vi "Pause.vi"(8 "error in (no error)":errorcluster, 11 "SSI PR Settings":T1) -> (0 "error out":errorcluster, 3 "SSI PR Settings":T1)   [LabVIEW 2018, in "SSI PR Pump.lvlib"]
uses:
  SSI PR Pump.lvlib
  SSI PR Settings Cluster.ctl
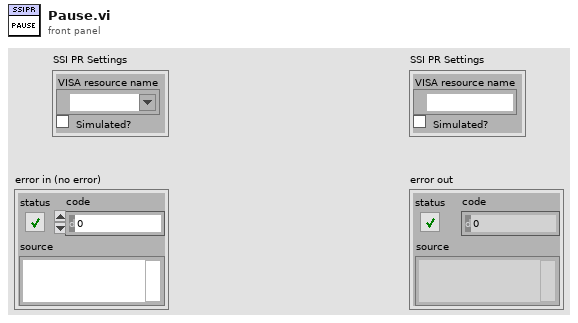
[diagram p1: front panel]
types:
  T1 = typedef "SSI PR Pump.lvlib/SSI PR Settings Cluster.ctl" = cluster{"VISA resource name":refnum<visa-resource-name>, "Simulated?":bool}
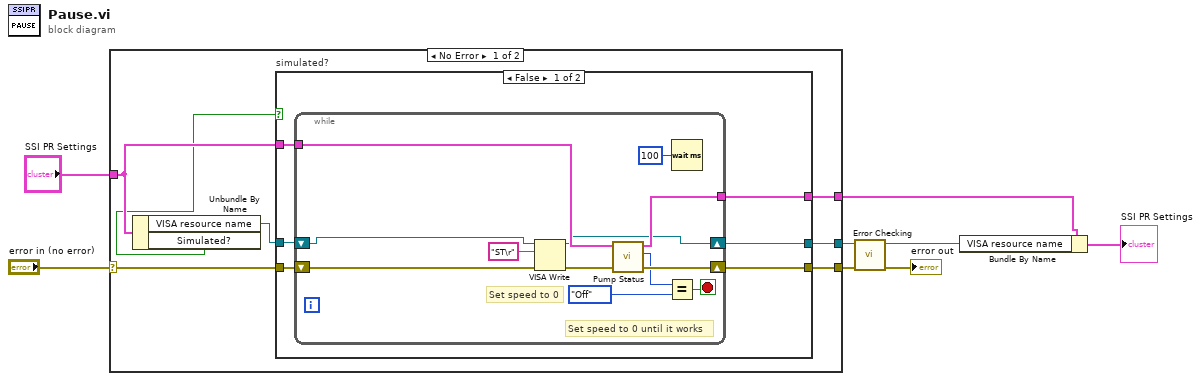
[diagram p0: block diagram]
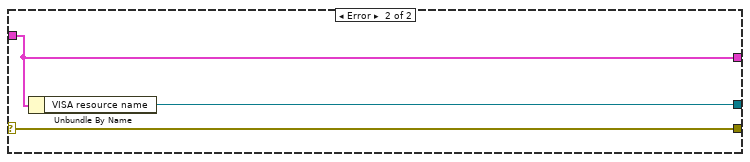
[diagram p3: hidden frame]
diagram:
  n1 = case shown="No Error" "error in (no error)" {
    selector: "error in (no error)" -> [w15 w39]
    tunnel: [w11 w38] -> w4
    tunnel: "SSI PR Settings" -> [w12 w38]
    tunnel: [w14 w37] -> w8
    tunnel: [w13 w39] -> w7
    frame No Error {
      n2 = Unbundle By Name(w12) -> ("VISA resource name"=w9:refnum<visa-resource-name>, "Simulated?"=w10:bool)
      n3 = case "simulated?" shown="False" w10 {
        tunnel: [w19 w36] -> w14
        tunnel: w9 -> [w21 w36]
        tunnel: w15 -> [w20 w35]
        tunnel: [w18 w35] -> w13
        tunnel: w12 -> [w17 w34]
        tunnel: [w16 w34] -> w11
        frame False {
          n4 = while {
            shift-right: [w23] -> w19
            shift-left: w21 -> [w33]
            shift-right: [w26] -> w18
            shift-left: w20 -> [w32]
            tunnel: w17 -> [w24]
            tunnel: [w25] -> w16
            stop <- w29 stop-if-true
            # "Set speed to 0 until it works"
            # "Set speed to 0"
            n5 = VISA Write(VISA resource name=w33, write buffer="ST\r" ("string"), error in (no error)=w32) -> (VISA resource name out=w23:refnum<visa-resource-name>, error out=w27:errorcluster)  [unwired: 1 out]
            n6 = call "Pump Status.vi"("error in (no error)"=w27, "SSI PR Settings"=w24) -> ("error out"=w26:errorcluster, "Pump On?"=w22:enum16{"Off", "On", "Not Initialized"}, "SSI PR Settings"=w25:T1)  [unwired: 5 in, 2 out]
            n7 = Equal?(x=w22, y=enum16{"Off", "On", "Not Initialized"}."Off") -> (x = y?=w29:bool)
            n8 = Wait (ms)(milliseconds to wait=u32 100) -> ()  [unwired: 1 out]
          }
        }
        frame True {
        }
      }
    }
    frame Error {
      n9 = Unbundle By Name(w38) -> ("VISA resource name"=w37:refnum<visa-resource-name>)
    }
  }
  n10 = call "Error Checking.vi"("error in (no error)"=w7, "VISA resource name"=w8) -> ("error out"=→"error out":errorcluster, "VISA resource name"=w6:refnum<visa-resource-name>)  [unwired: 7 in, 1 out]
  n11 = Bundle By Name(cluster=w4, "VISA resource name"=w6) -> (→"SSI PR Settings":T1)
